vi "Init MCP.vi"(8 "error in (no error)":errorcluster, 11 "Data Cluster in":T1) -> (0 "error out":errorcluster, 3 "Data Cluster out":T1)   [LabVIEW 2020, in "G-AI Core.lvlib"]
uses:
  G-AI Core.lvlib
  Module Data--cluster.ctl
  <vilib>/jgoebel/LabVIEW MCP Server SDK/src/MCP Server/jg_mcp_MCP Server.lvlib
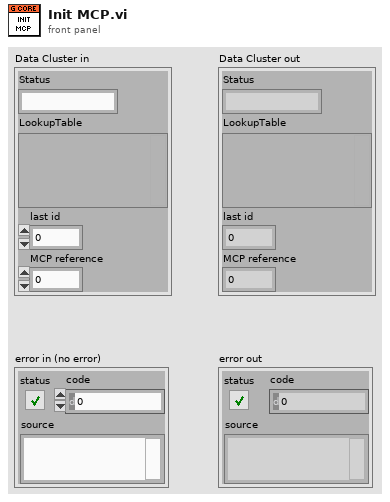
[diagram p1: front panel]
types:
  T1 = typedef "G-AI Core.lvlib/Module Data--cluster.ctl" = cluster{"Status":string, "LookupTable":variant, "last id":i32, "MCP reference":i32}
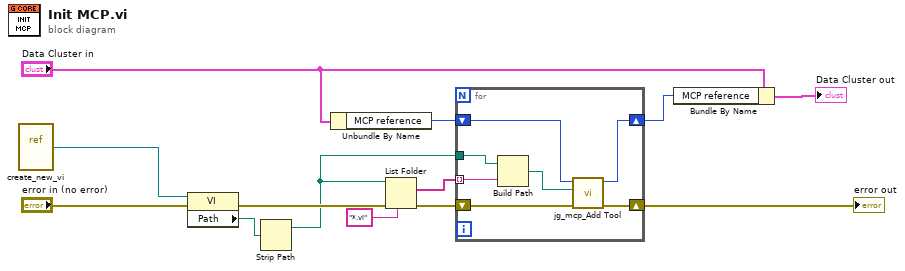
[diagram p0: block diagram]
diagram:
  n1 = vi-ref "create_new_vi.vi"() -> (w3:refnum<vi>)
  n2 = property class="VI"(reference=w3, error in="error in (no error)") -> (error out=w4:errorcluster, "Path"=w2:path)  [unwired: 1 out]
  n3 = Strip Path(path=w2) -> (stripped path=w1:path)  [unwired: 1 out]
  n4 = Unbundle By Name("Data Cluster in") -> ("MCP reference"=w11:i32)
  n5 = List Folder(path=w1, pattern="*.vi", error in=w4) -> (filenames=w7:string[], error out=w8:errorcluster)  [unwired: 1 in, 2 out]
  n6 = for {
    shift-right: [w20] -> w12
    shift-left: w8 -> [w18]
    tunnel: w1 -> [w17]
    tunnel: w7 -> [w16] mode=indexing
    shift-right: [w14] -> w5
    shift-left: w11 -> [w19]
    n7 = Build Path(base path=w17, name or relative path=w16) -> (appended path=w15:path)
    n8 = call <vilib>:"jg_mcp_Add Tool.vi"("error in (no error)"=w18, "vi path"=w15, "server id"=w19) -> ("error out"=w20:errorcluster, "server id out"=w14:i32)  [unwired: 7 in]
  }
  "error out" <- w12
  n9 = Bundle By Name(cluster="Data Cluster in", "MCP reference"=w5) -> (→"Data Cluster out":T1)
